vi "双路双通通断器（SGL）.vi"(7 "默认值":sgl=nan, 9 "直通？":bool=TRUE, 10 "Y_In":sgl, 11 "X_In":sgl) -> (2 "Y_Out":sgl, 3 "X_Out":sgl)   [LabVIEW 2011]
doc: "功能：\n\n返回一个枚举，表明输入数的范围，用于三段比较。\n\n\nCSXCS_366创建。"
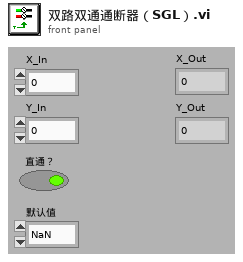
[diagram p1: front panel]
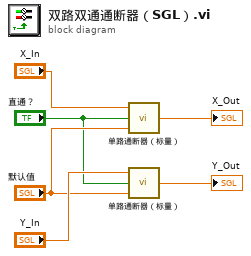
[diagram p0: block diagram]
diagram:
  n1 = call-poly "单路通断器（标量）.vi"("默认值"="默认值", "直通？"="直通？", "X_In"="X_In") -> ("X_Out"=→"X_Out":sgl)
  n2 = call-poly "单路通断器（标量）.vi"("默认值"="默认值", "直通？"="直通？", "X_In"="Y_In") -> ("X_Out"=→"Y_Out":sgl)
